vi "Main_2.vi"() -> ()   [LabVIEW 2013]
doc: "Use this template to build a simple state machine design pattern. Each state executes code and determines which state to transition to."
uses:
  controls/Data.ctl
  controls/State.ctl
panel:
  in  "Feeder Input":i16=1
  in  "Corridor Input":i16=2
  out "refnum out":refnum<k1>
  in  "Feeder Delay":u32=500
  in  "Corridor Delay":u32=500
  in  "Sample Delay":i32=50
  out "Data":T1
  out "Beam":u32
  in  "@Feeder":bool
  in  "Feeder Enable":bool
  in  "EoCo":bool
  in  "Exit":bool
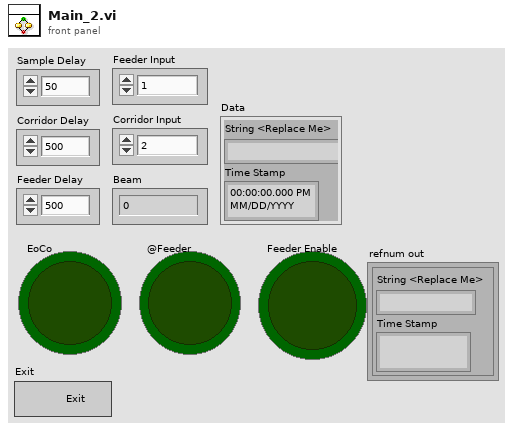
[diagram p1: front panel]
types:
  T1 = typedef "Data.ctl" = cluster{"String <Replace Me>":string, "Time Stamp":timestamp}
  T2 = typedef "State.ctl" = enum16{"Initialize", "Refresh", "Wait for Event", "End of Corridor", "End of Corridor Delay", "Feed", "Feed Delay", "Exit"}
  T3 = enum16{"open", "replace", "create", "open or create", "replace or create", "replace or create with confirmation"}
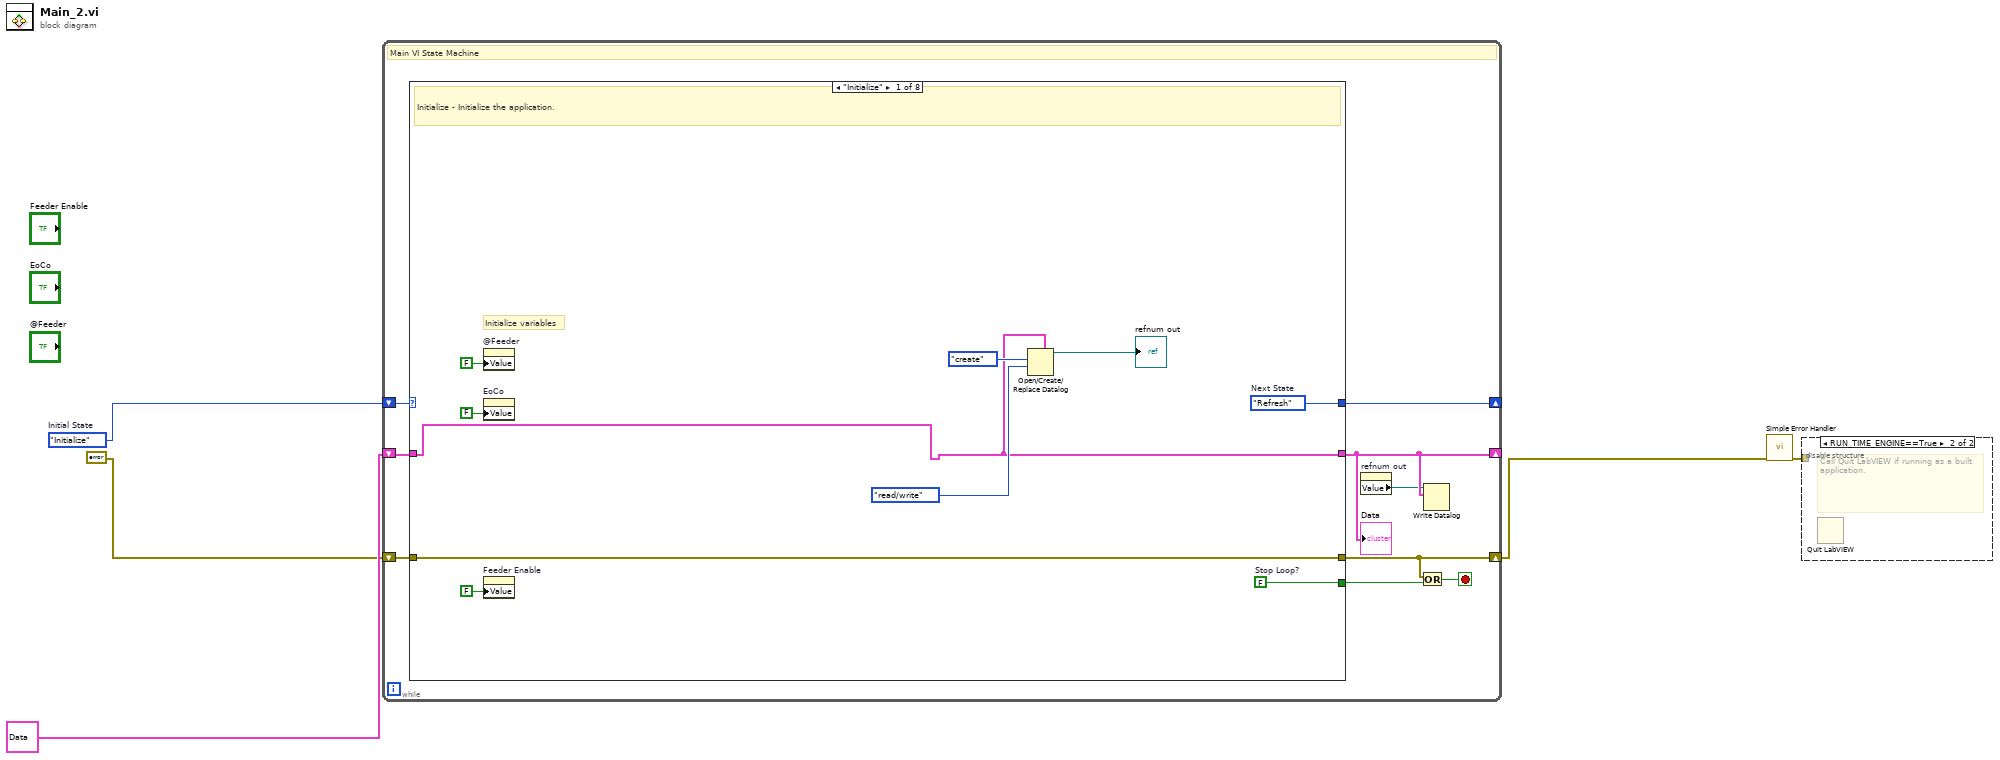
[diagram p0: block diagram]
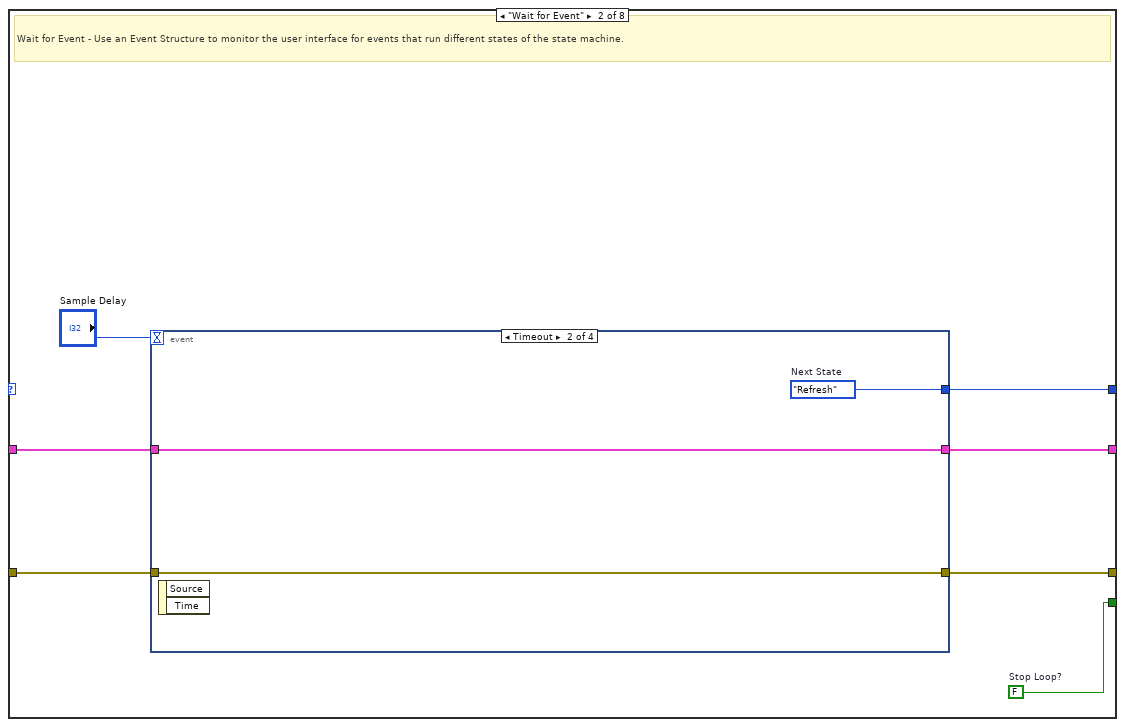
[diagram p3: hidden frame]
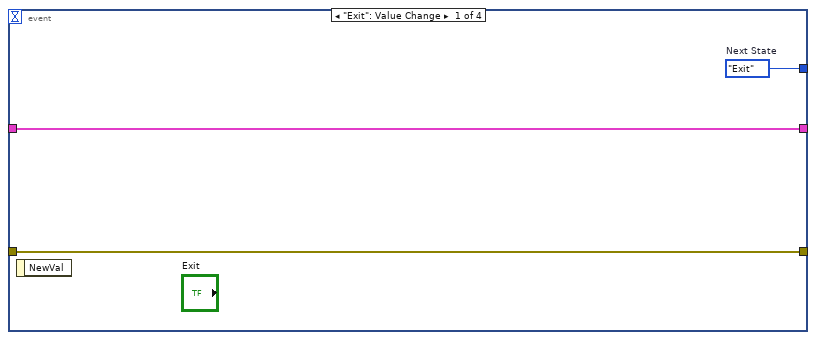
[diagram p4: hidden frame]
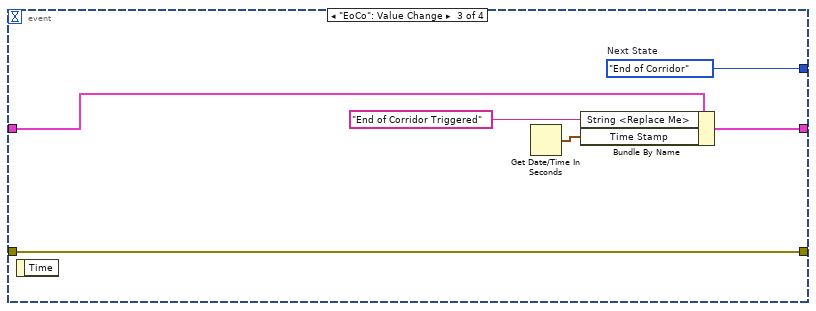
[diagram p5: hidden frame]
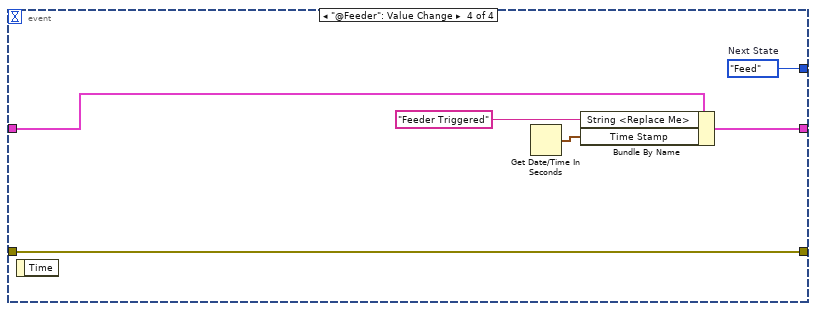
[diagram p6: hidden frame]
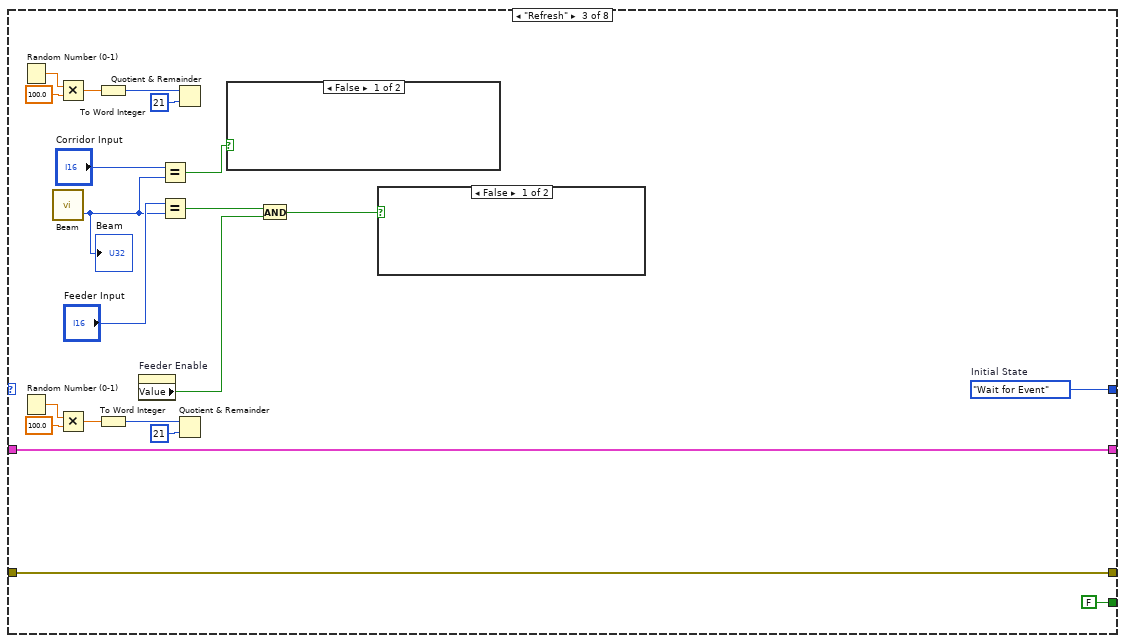
[diagram p7: hidden frame]
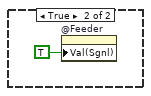
[diagram p8: hidden frame]
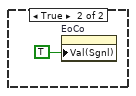
[diagram p9: hidden frame]
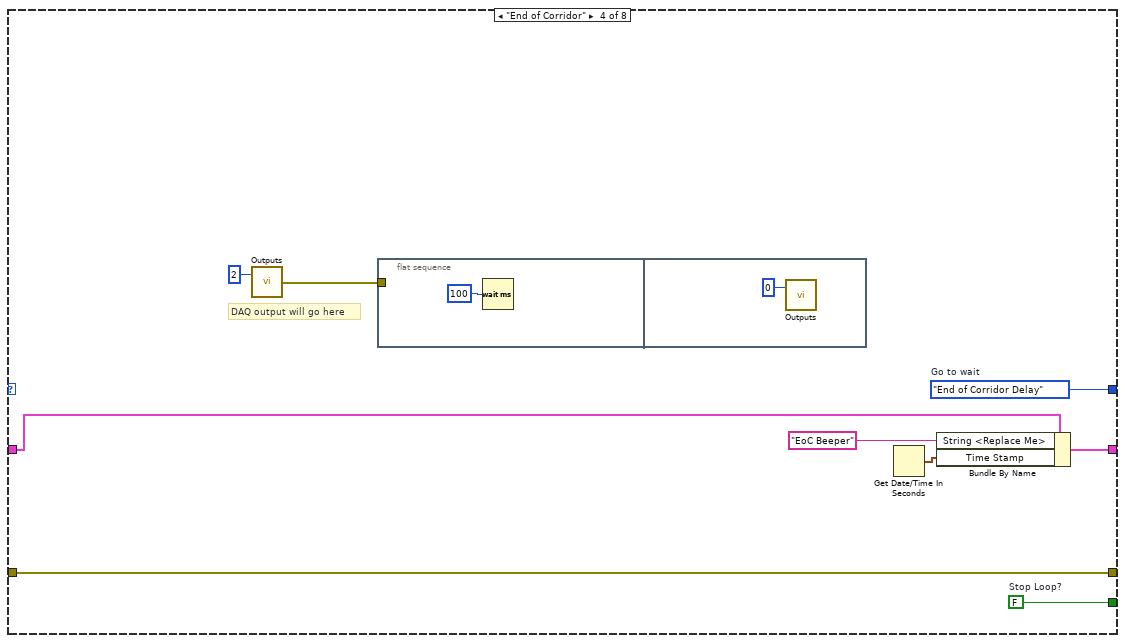
[diagram p10: hidden frame]
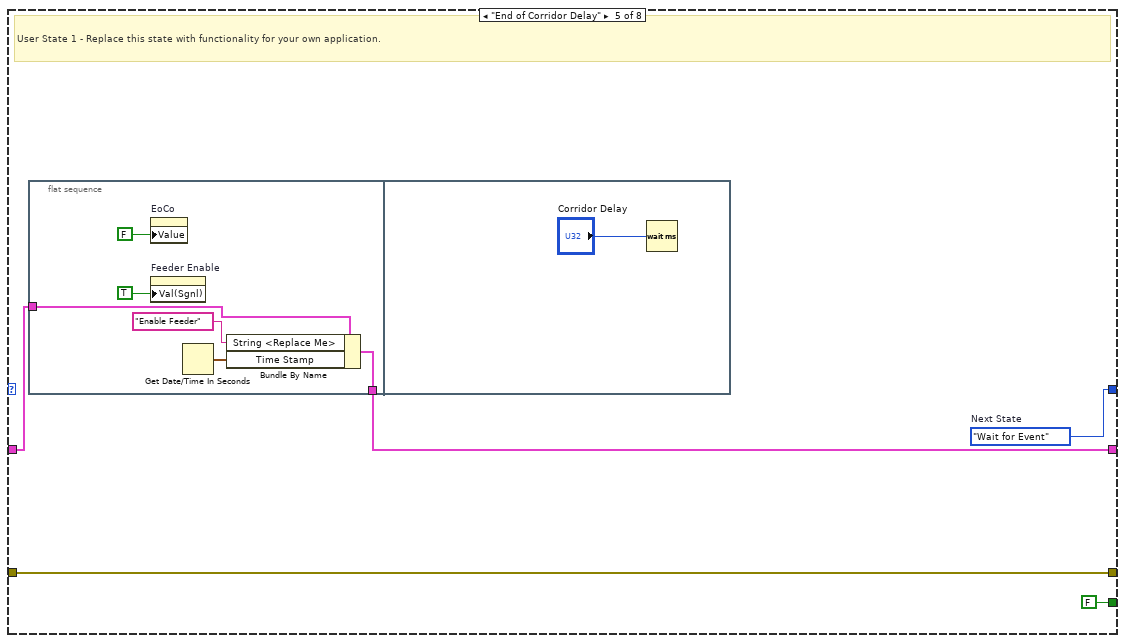
[diagram p11: hidden frame]
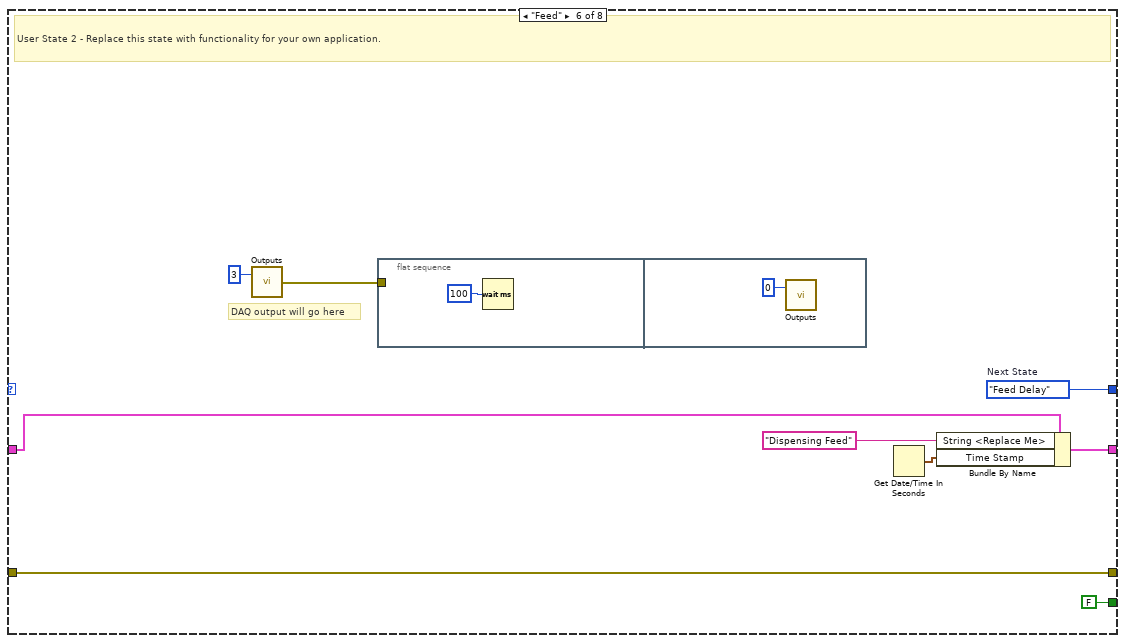
[diagram p12: hidden frame]
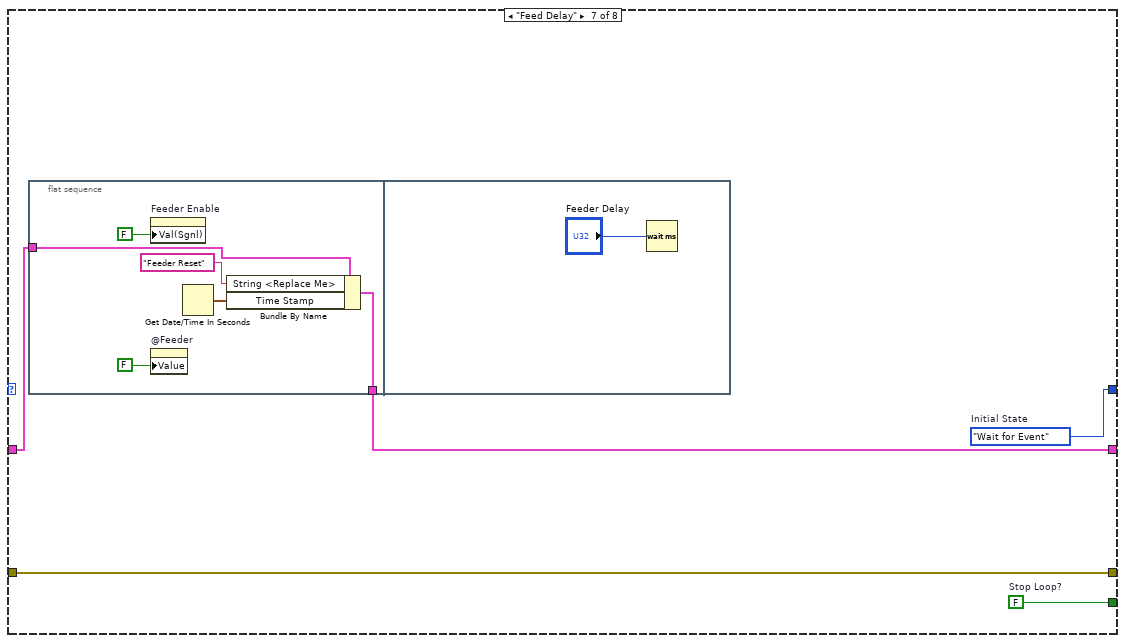
[diagram p13: hidden frame]
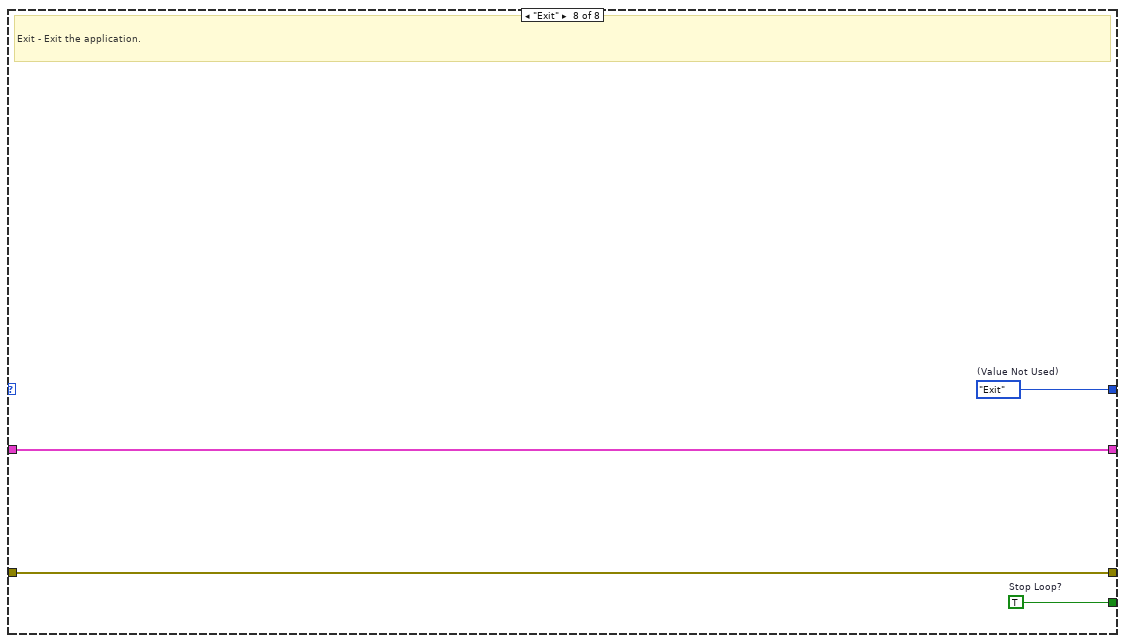
[diagram p14: hidden frame]
diagram:
  w5 = State."Initialize"  # Initial State
  n1 = while {
    shift-right: [w13] -> _
    shift-left: w5 -> [w14]
    shift-right: [w7] -> _
    shift-left: T1 {"String <Replace Me>"="", "Time Stamp"=timestamp(0 s since 1904-01-01)} ("Data") -> [w12]
    shift-right: [w8] -> w2
    shift-left: errorcluster {"status"=FALSE, "code"=0, "source"=""} ("error constant") -> [w11]
    stop <- w9 stop-if-true
    # "Main VI State Machine"
    n2 = case shown="\"Initialize\"" w14 {
      tunnel: [w24 w31 w68 w80 w88 w104 w110 w122] -> w13
      tunnel: [w23 w30 FALSE ("Stop Loop?") w79 FALSE ("Stop Loop?") FALSE ("Stop Loop?") w109 w119] -> w10
      tunnel: w12 -> [w15 w29 w70 w74 w85 w99 w108 w121]
      tunnel: [w15 w28 w70 w73 w84 w98 w107 w121] -> w7
      tunnel: w11 -> [w22 w27 w69 w81 w86 w102 w111 w120]
      tunnel: [w22 w26 w69 w81 w86 w102 w111 w120] -> w8
      frame "Initialize" {
        w23 = FALSE  # Stop Loop?
        w24 = State."Refresh"  # Next State
        # "Initialize variables"
        # "Initialize - Initialize the application."
        n3 = property on="@Feeder" class="Bool (strict)"("Value"=FALSE ("@Feeder")) -> ()  [unwired: 2 in, 2 out]
        n4 = property on="EoCo" class="Bool (strict)"("Value"=FALSE ("Value (Signaling)")) -> ()  [unwired: 2 in, 2 out]
        n5 = property on="Feeder Enable" class="Bool (strict)"("Value"=FALSE) -> ()  [unwired: 2 in, 2 out]
        n6 = Open/Create/Replace Datalog(5:w15, 9:enum16{"read/write", "read-only", "write-only"}."read/write" ("access (0:read/write)"), 10:T3."create" ("operation (0:open)")) -> (3:→"refnum out":refnum<k1>)  [unwired: 3 in, 2 out]
      }
      frame "Wait for Event" {
        w30 = FALSE  # Stop Loop?
        # "Wait for Event - Use an Event Structure to monitor the user interface for events that run different states of the state machine."
        n7 = event shown="[1] Timeout" {
          selector: _ -> [_ _ _ _]
          dyn-events: _ -> [_ _ _ _]
          timeout: "Sample Delay" -> [_ _ _ _]
          tunnel: [w34 w36 w43 w49] -> w31
          tunnel: w29 -> [w33 w35 w42 w48]
          tunnel: [w33 w35 w41 w47] -> w28
          tunnel: w27 -> [w32 w37 w39 w45]
          tunnel: [w32 w37 w39 w45] -> w26
          event "Exit": Value Change {
            w34 = State."Exit"  # Next State
            n8 = event-data() -> ()  [unwired: 1 in, 1 out]
          }
          event Timeout {
            w36 = State."Refresh"  # Next State
            n9 = event-data() -> ()  [unwired: 1 in, 2 out]
          }
          event "EoCo": Value Change {
            w43 = State."End of Corridor"  # Next State
            n10 = event-data() -> ()  [unwired: 1 in, 1 out]
            n11 = Get Date/Time In Seconds() -> (seconds since 1Jan1904=w38:timestamp)
            n12 = Bundle By Name(cluster=w42, "String <Replace Me>"="End of Corridor Triggered" ("Running User State 1"), "Time Stamp"=w38) -> (w41:T1)
          }
          event "@Feeder": Value Change {
            w49 = State."Feed"  # Next State
            n13 = event-data() -> ()  [unwired: 1 in, 1 out]
            n14 = Get Date/Time In Seconds() -> (seconds since 1Jan1904=w44:timestamp)
            n15 = Bundle By Name(cluster=w48, "String <Replace Me>"="Feeder Triggered" ("Running User State 2"), "Time Stamp"=w44) -> (w47:T1)
          }
        }
      }
      frame "Refresh" {
        w68 = State."Wait for Event"  # Initial State
        n16 = Random Number (0-1)() -> (number: 0 to 1=w56:dbl)
        n17 = Random Number (0-1)() -> (number: 0 to 1=w63:dbl)
        n18 = call "Beam.vi"() -> ("return type"=w50:i16)  [unwired: 1 in, 1 out]
        "Beam" <- w50
        n19 = Multiply(x=w56, y=100.0) -> (x*y=w57:dbl)
        n20 = Multiply(x=w63, y=100.0) -> (x*y=w62:dbl)
        n21 = To Word Integer(number=w57) -> (16bit integer=w58:i16)
        n22 = To Word Integer(number=w62) -> (16bit integer=w65:i16)
        n23 = property on="Feeder Enable" class="Bool (strict)"() -> ("Value"=w67:bool)  [unwired: 2 in, 2 out]
        n24 = Equal?(x="Corridor Input", y=w50) -> (x = y?=w59:bool)
        n25 = Equal?(x="Feeder Input", y=w50) -> (x = y?=w60:bool)
        n26 = Quotient & Remainder(x=w58, y=u32 21) -> ()  [unwired: 2 out]
        n27 = Quotient & Remainder(x=w65, y=i16 21) -> ()  [unwired: 2 out]
        n28 = case shown="False" w59 {
          frame False {
          }
          frame True {
            n29 = property on="EoCo" class="Bool (strict)"("Val(Sgnl)"=TRUE ("Value (Signaling)")) -> ()  [unwired: 2 in, 2 out]
          }
        }
        n30 = And(x=w60, y=w67) -> (x .and. y?=w61:bool)
        n31 = case shown="False" w61 {
          frame False {
          }
          frame True {
            n32 = property on="@Feeder" class="Bool (strict)"("Val(Sgnl)"=TRUE ("Value (Signaling)")) -> ()  [unwired: 2 in, 2 out]
          }
        }
      }
      frame "End of Corridor" {
        w79 = FALSE  # Stop Loop?
        w80 = State."End of Corridor Delay"  # Go to wait
        # "DAQ output will go here"
        n33 = call "Outputs.vi"("Value"=i16 2) -> ("error out"=w78:errorcluster)  [unwired: 1 in]
        n34 = flat-sequence {
          tunnel: w78 -> [_]
          frame #0 {
            n35 = Wait (ms)(milliseconds to wait=u32 100) -> ()  [unwired: 1 out]
          }
          frame #1 {
            n36 = call "Outputs.vi"("Value"=i16 0) -> ()  [unwired: 1 in, 1 out]
          }
        }
        n37 = Get Date/Time In Seconds() -> (seconds since 1Jan1904=w75:timestamp)
        n38 = Bundle By Name(cluster=w74, "String <Replace Me>"="EoC Beeper", "Time Stamp"=w75) -> (w73:T1)
      }
      frame "End of Corridor Delay" {
        w88 = State."Wait for Event"  # Next State
        # "User State 1 - Replace this state with functionality for your own application."
        n39 = flat-sequence {
          tunnel: w85 -> [w90]
          tunnel: [w89] -> w84
          frame #0 {
            n40 = property on="EoCo" class="Bool (strict)"("Value"=FALSE ("Value (Signaling)")) -> ()  [unwired: 2 in, 2 out]
            n41 = property on="Feeder Enable" class="Bool (strict)"("Val(Sgnl)"=TRUE ("Value (Signaling)")) -> ()  [unwired: 2 in, 2 out]
            n42 = Get Date/Time In Seconds() -> (seconds since 1Jan1904=w92:timestamp)
            n43 = Bundle By Name(cluster=w90, "String <Replace Me>"="Enable Feeder", "Time Stamp"=w92) -> (w89:T1)
          }
          frame #1 {
            n44 = Wait (ms)(milliseconds to wait="Corridor Delay") -> ()  [unwired: 1 out]
          }
        }
      }
      frame "Feed" {
        w104 = State."Feed Delay"  # Next State
        # "DAQ output will go here"
        # "User State 2 - Replace this state with functionality for your own application."
        n45 = call "Outputs.vi"("Value"=i16 3) -> ("error out"=w101:errorcluster)  [unwired: 1 in]
        n46 = flat-sequence {
          tunnel: w101 -> [_]
          frame #0 {
            n47 = Wait (ms)(milliseconds to wait=u32 100) -> ()  [unwired: 1 out]
          }
          frame #1 {
            n48 = call "Outputs.vi"("Value"=i16 0) -> ()  [unwired: 1 in, 1 out]
          }
        }
        n49 = Get Date/Time In Seconds() -> (seconds since 1Jan1904=w97:timestamp)
        n50 = Bundle By Name(cluster=w99, "String <Replace Me>"="Dispensing Feed", "Time Stamp"=w97) -> (w98:T1)
      }
      frame "Feed Delay" {
        w109 = FALSE  # Stop Loop?
        w110 = State."Wait for Event"  # Initial State
        n51 = flat-sequence {
          tunnel: w108 -> [w113]
          tunnel: [w112] -> w107
          frame #0 {
            n52 = property on="Feeder Enable" class="Bool (strict)"("Val(Sgnl)"=FALSE ("Value (Signaling)")) -> ()  [unwired: 2 in, 2 out]
            n53 = property on="@Feeder" class="Bool (strict)"("Value"=FALSE ("@Feeder")) -> ()  [unwired: 2 in, 2 out]
            n54 = Get Date/Time In Seconds() -> (seconds since 1Jan1904=w114:timestamp)
            n55 = Bundle By Name(cluster=w113, "String <Replace Me>"="Feeder Reset", "Time Stamp"=w114) -> (w112:T1)
          }
          frame #1 {
            n56 = Wait (ms)(milliseconds to wait="Feeder Delay") -> ()  [unwired: 1 out]
          }
        }
      }
      frame "Exit" {
        w119 = TRUE  # Stop Loop?
        w122 = State."Exit"  # (Value Not Used)
        # "Exit - Exit the application."
      }
    }
    "Data" <- w7
    n57 = property on="refnum out" class="TypRef (strict)"() -> ("Value"=w6:refnum<k1>)  [unwired: 2 in, 2 out]
    n58 = Or(x=w8, y=w10) -> (x .or. y?=w9:bool)
    n59 = Write Datalog(6:w7, 7:w6) -> ()  [unwired: 1 in, 2 out]
  }
  n60 = call <vilib>:"Simple Error Handler.vi"("error in (no error)"=w2) -> ("error out"=w1:errorcluster)  [unwired: 4 in, 4 out]
  n61 = disable-structure shown="RUN_TIME_ENGINE==True" {
    disable-tunnel: w1 -> [_ _]
    frame condition #0 (active) {
    }
    frame condition #1 {
      # "Call Quit LabVIEW if running as a built application."
      n62 = Quit LabVIEW() -> ()  [unwired: 1 in]
    }
  }
